vi "AlazarInputControl.vi"(0 "Handle":u64, 1 "Channel":u8(ring)=1 items=["A"=1, "B"=2, "C"=4, "D"=8], 2 "Coupling":u32(ring)=2 items=["AC"=1, "DC"=2], 3 "Range":u32(ring)=10 items=["20 mV"=1, "40 mV"=2, "50 mV"=3, "80 mV"=4, "100 mV"=5, "200 mV"=6, "400 mV"=7, "500 mV"=8, "800 mV"=9, "1 V"=10, "1.25 V"=33, "2 V"=11, "4 V"=12, "5 V"=13, "8 V"=14, "10 V"=15, "20 V"=16], 4 "Impedance":u32(ring)=2 items=["1 MOhm"=1, "50 Ohm"=2, ""=0], 5 "error in (no error)":errorcluster) -> (14 "Handle":u64, 18 "Return Code":u32, 19 "error out":errorcluster)   [LabVIEW 2018]
doc: "Select the input coupling, range, and impedance of a digitizer channel."
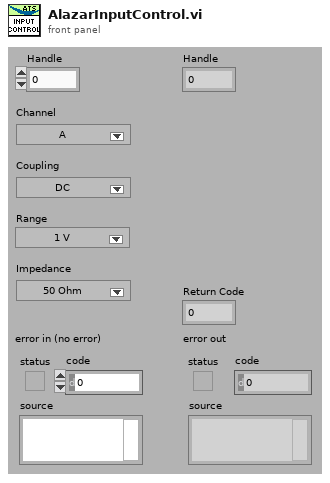
[diagram p1: front panel]
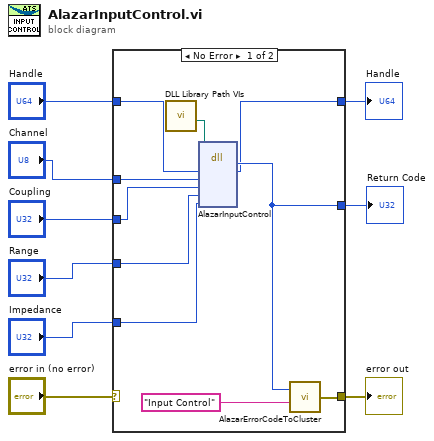
[diagram p0: block diagram]
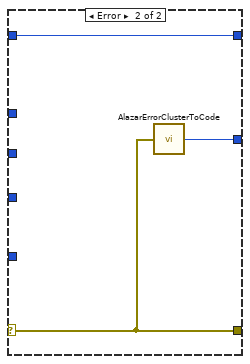
[diagram p2: hidden frame]
diagram:
  n1 = case shown="No Error" "error in (no error)" {
    selector: "error in (no error)" -> [_ w22]
    tunnel: [w16 w22] -> w8
    tunnel: [w18 w21] -> w7
    tunnel: "Handle" -> [w19 w20]
    tunnel: [w15 w20] -> w5
    tunnel: "Coupling" -> [w12 _]
    tunnel: "Range" -> [w13 _]
    tunnel: "Impedance" -> [w14 _]
    tunnel: "Channel" -> [w11 _]
    frame No Error {
      n2 = call "DLL Library Path VIs.vi"() -> ("Alazar"=w10:path)  [unwired: 4 in, 7 out]
      n3 = dll-call lib="C:/Project/SerialSectOCT - FFT GPU/SerialSectOCT/Labview Software/DLL/ATSApi.dll" fn="AlazarInputControl"(path in=w10, "handle"=w19, "channelID"=w11, "couplingID"=w12, "rangeID"=w13, "ImpedanceID"=w14) -> ("return type"=w18:u32, "handle"=w15:u64)  [unwired: 6 in, 2 out]
      n4 = call "AlazarErrorCodeToCluster.vi"("Message"="Input Control", "Error Code"=w18) -> ("error out"=w16:errorcluster)
    }
    frame Error {
      n5 = call "AlazarErrorClusterToCode.vi"("error in (no error)"=w22) -> ("Error Code"=w21:u32)
    }
  }
  "Handle" <- w5
  "error out" <- w8
  "Return Code" <- w7
